vi "trace_data.vi"(8 "error in":errorcluster, 11 "Decimate":i32=1) -> (0 "error out":errorcluster, 2 "Trace timestamp":timestamp, 3 "Decimated trace":sgl[][][](array[numeric]) format="%#_5g")   [LabVIEW 2013]
panel:
  # "If -1, decimate to single point."
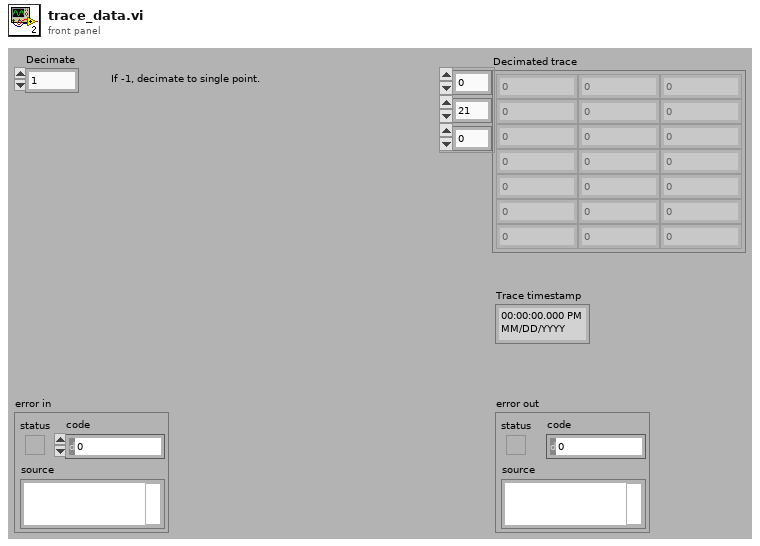
[diagram p1: front panel]
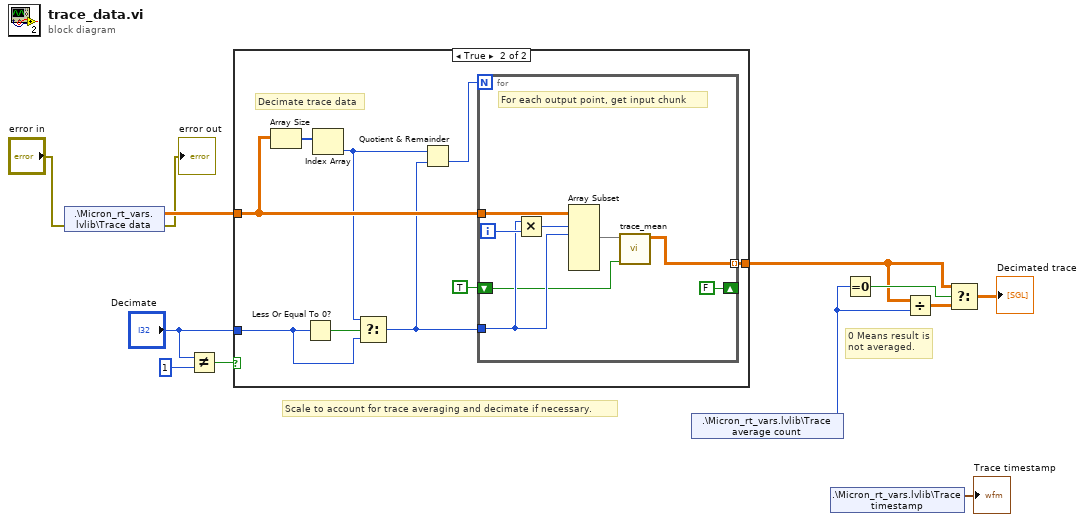
[diagram p0: block diagram]
diagram:
  # "0 Means result is not averaged."
  # "Scale to account for trace averaging and decimate if necessary."
  n1 = shared-variable ".\\Micron_rt_vars.lvlib\\Trace data"(error in="error in") -> (w9:sgl[][][], error out=→"error out":errorcluster)
  n2 = Not Equal?(x="Decimate", y=1) -> (x != y?=w10:bool)
  n3 = case shown="True" w10 {
    tunnel: "Decimate" -> [_ w15]
    tunnel: [w13 w20] -> w5
    tunnel: w9 -> [w13 w21]
    frame False {
      # "No decimation"
    }
    frame True {
      # "Decimate trace data"
      n4 = Array Size(array=w21) -> (size(s)=w22:i32[])
      n5 = Less Or Equal To 0?(x=w15) -> (x <= 0?=w19:bool)
      n6 = Index Array(array=w22) -> (element=w18:i32)  [unwired: 1 in]
      n7 = Select(t=w18, s=w19, f=w15) -> (s? t:f=w17:i32)
      n8 = Quotient & Remainder(x=w18, y=w17) -> (floor(x/y)=w16:i32)  [unwired: 1 out]
      n9 = for {
        N: w16 -> [_]
        tunnel: w21 -> [w27]
        tunnel: w17 -> [w28]
        tunnel: [w26] -> w20 mode=indexing
        shift-right: [FALSE] -> _
        shift-left: TRUE -> [w24]
        i -> [w30]
        # "For each output point, get input chunk"
        n10 = Multiply(x=w28, y=w30) -> (x*y=w29:i32)
        n11 = Array Subset(array=w27, index (dim 0)=w29, length (dim 0)=w28) -> (w25:sgl[][][])  [unwired: 4 in]
        n12 = call "trace_mean.vi"("Reset"=w24, "Array in"=w25) -> ("Array out"=w26:sgl[][])  [unwired: 9 in]
      }
    }
  }
  n13 = shared-variable ".\\Micron_rt_vars.lvlib\\Trace average count"() -> (w8:u32)  [unwired: 2 out]
  n14 = shared-variable ".\\Micron_rt_vars.lvlib\\Trace timestamp"() -> (→"Trace timestamp":timestamp)  [unwired: 1 in, 1 out]
  n15 = Equal To 0?(x=w8) -> (x = 0?=w6:bool)
  n16 = Divide(x=w5, y=w8) -> (x/y=w7:sgl[][][])
  n17 = Select(t=w5, s=w6, f=w7) -> (s? t:f=→"Decimated trace":sgl[][][])
